vi "Create Init Test Configuration.vi"(8 "error in":errorcluster, 10 "Connection Configuration":T2={"Client?"=FALSE, "Server Certificates"={"Relative Path?"=FALSE, "Certificate Paths"=[], "Certificate Names"=[]}, "Client Certificates"={"Relative Path?"=FALSE, "Certificate Paths"=[], "Certificate Names"=[]}, "Client Configuration"={"Server Endpoint URL"="", "Security Policy"={"Message Mode"=enum."None", "Security"=enum."Basic256"}, "Username/Password"={"Username"="", "Password"=""}}, "Server Configuration"={"Server Name"="", "TCP port (49580)"="49580", "Supported Security Policies"={"None"=TRUE, "Sign with Basic128Rsa125"=FALSE, "Sign and Encrypt with Basic128Rsa125"=FALSE, "Sign with Basic256"=FALSE, "Sign and Encrypt with Basic256"=FALSE}}}) -> (0 "error out":errorcluster, 3 "module":refnum<class "OPC UA configuration.lvclass">)   [LabVIEW 2013, in "OPC UA tests.lvlib"]
doc: "This VI creates the test configuration used in testing. BY default just creates one line with every datatype"
uses:
  OPC UA tests.lvlib
  module/configuration/OPC UA configuration.lvclass
  <vilib>/OPCUA/server/subVI/supported security policies.ctl
  <vilib>/NI/Tag Bus Module Framework/channel/channel classification.ctl
  module/configuration/OPC UA Data Type.ctl
  module/configuration/Line.ctl
  <vilib>/NI/Tag Bus Module Framework/channel/TBM channel.lvclass
  module/configuration/OPC UA configuration.lvclass/OPC UA configuration.ctl
  module/configuration/Write Connection Configuration.vi
  <vilib>/NI/Configuration Framework/serializable configuration/NISE_CEF_serializable configuration.lvclass
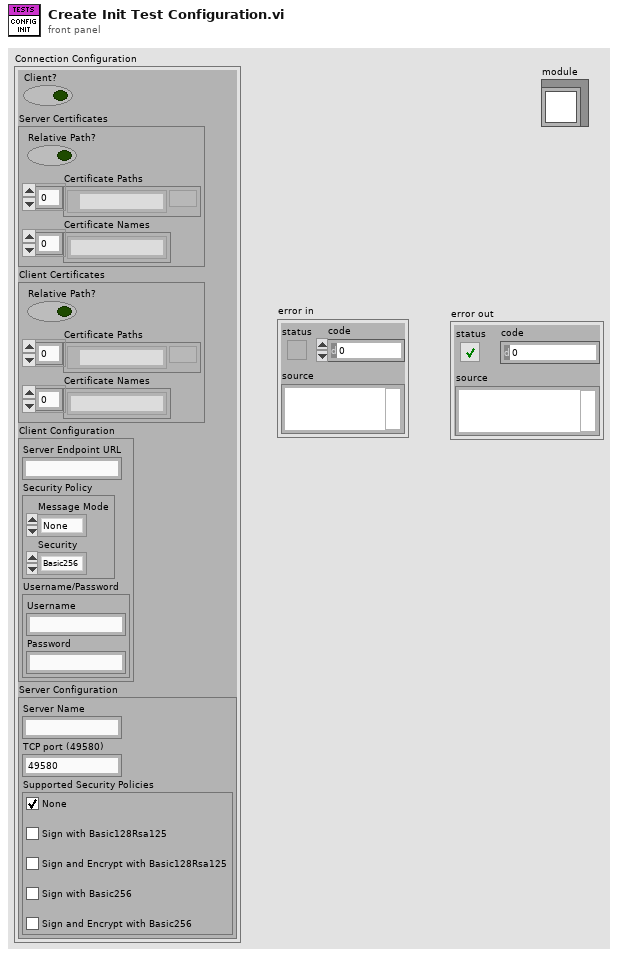
[diagram p1: front panel]
types:
  T1 = typedef "supported security policies.ctl" = cluster{"None":bool, "Sign with Basic128Rsa125":bool, "Sign and Encrypt with Basic128Rsa125":bool, "Sign with Basic256":bool, "Sign and Encrypt with Basic256":bool}
  T2 = cluster{"Client?":bool, "Server Certificates":cluster{"Relative Path?":bool, "Certificate Paths":path[], "Certificate Names":string[]}, "Client Certificates":cluster{"Relative Path?":bool, "Certificate Paths":path[], "Certificate Names":string[]}, "Client Configuration":cluster{"Server Endpoint URL":string, "Security Policy":cluster{"Message Mode":enum16{"None", "Sign", "Sign and Encrypt"}, "Security":enum16{"Basic256", "Basic128Rsa15"}}, "Username/Password":cluster{"Username":string, "Password":string}}, "Server Configuration":cluster{"Server Name":string, "TCP port (49580)":string, "Supported Security Policies":T1}}
  T3 = typedef "TBM channel.lvclass/channel classification.ctl" = enum16{"input data", "output data", "processing parameter", "processing result"}
  T4 = typedef "OPC UA configuration.lvclass/OPC UA Data Type.ctl" = u16
  T5 = typedef "OPC UA configuration.lvclass/Line.ctl" = cluster{"channel":refnum<class "TBM channel.lvclass">, "Node Path":string, "OPC UA Data Type":T4}
  T6 = typedef "tag bus.lvlib/tag descriptor.lvclass/Data Type.ctl" = enum16{"Double", "Single", "I64", "I32", "I16", "I8", "U64", "U32", "U16", "U8", "Boolean", "String", "Array of Double", "Array of Single", "Array of I64", "Array of I32", "Array of I16", "Array of I8", "Array of U64", "Array of U32", "Array of U16", "Array of U8", "Array of Boolean", "Array of String"}
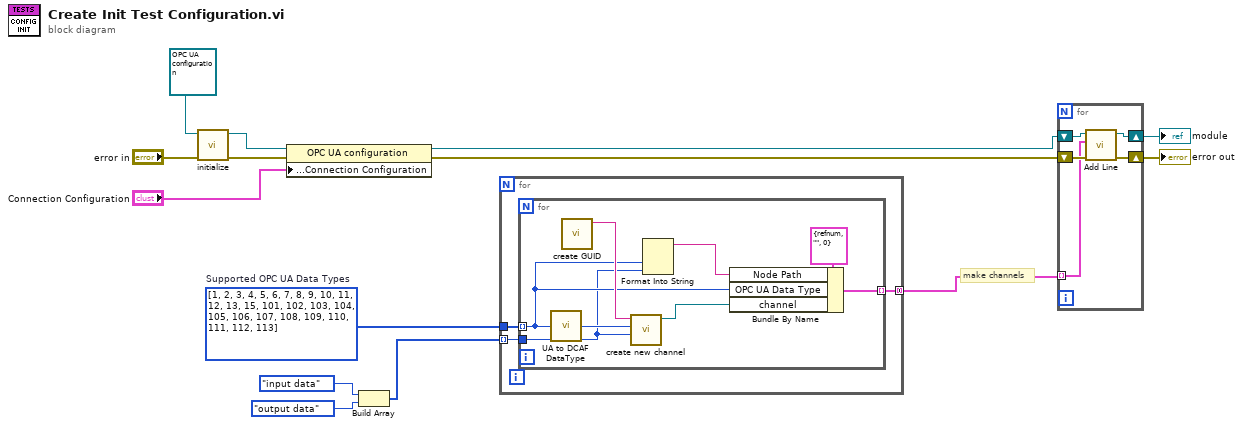
[diagram p0: block diagram]
diagram:
  w5 = T4[] [1, 2, 3, 4, 5, 6, 7, 8, 9, 10, 11, 12, 13, 15, 101, 102, 103, 104, 105, 106, 107, 108, 109, 110, 111, 112, 113] items=["Boolean"=1, "SByte"=2, "Byte"=3, "Int16"=4, "UInt16"=5, "Int32"=6, "UInt32"=7, "Int64"=8, "UInt64"=9, "Float"=10, "Double"=11, "String"=12, "DateTime"=13, "ByteString"=15, "Array of Boolean"=101, "Array of SByte"=102, "Array of Byte"=103, "Array of Int16"=104, "Array of UInt16"=105, "Array of Int32"=106, "Array of UInt32"=107, "Array of Int64"=108, "Array of UInt64"=109, "Array of Float"=110, "Array of Double"=111, "Array of String"=112, "Array of DateTime"=113, "Array of ByteString"=115]  # Supported OPC UA Data Types
  # "make channels"
  n1 = call <vilib>:"initialize.vi"("error in"="error in", "configuration in"=refnum<class "OPC UA configuration.lvclass"> refnum ("tag bus configurable plugin module configuration")) -> ("error out"=w13:errorcluster, "configuration out"=w11:refnum<class "OPC UA configuration.lvclass">)  [unwired: 7 in, 1 out]
  n2 = property class="OPC UA configuration"(reference=w11, error in=w13, "Customize:Properties:Connection Configuration"="Connection Configuration") -> (reference out=w7:refnum<class "OPC UA configuration.lvclass">, error out=w12:errorcluster)
  n3 = Build Array(channel_classification."input data" ("channel classification"), channel_classification."output data" ("channel classification")) -> (w2:T3[])
  n4 = for {
    tunnel: [w17] -> w10 mode=concatenating
    tunnel: w5 -> [w16]
    tunnel: w2 -> [w15] mode=indexing
    n5 = for {
      tunnel: [w23] -> w17 mode=indexing
      tunnel: w16 -> [w19] mode=indexing
      tunnel: w15 -> [w18]
      n6 = call "UA to DCAF DataType.vi"("OPC UA Data Type"=w19) -> ("DCAF Datatype"=w21:T6)
      n7 = call <vilib>:"create GUID.vi"() -> ("uuid"=w25:string)  [unwired: 10 in, 1 out]
      n8 = call <vilib>:"create new channel.vi"("channel classification"=w18, "data type"=w21, "channel name"=w25) -> ("channel"=w22:refnum<class "TBM channel.lvclass">)  [unwired: 8 in]
      n9 = Format Into String(w19, w18) -> (resulting string=w20:string)  [unwired: 3 in, 1 out]
      n10 = Bundle By Name(cluster=T5 {"channel"=refnum, "Node Path"="", "OPC UA Data Type"=0} ("Line"), "Node Path"=w20, "OPC UA Data Type"=w19, "channel"=w22) -> (w23:T5)
    }
  }
  n11 = for {
    tunnel: w10 -> [w26] mode=indexing
    shift-right: [w29] -> w9
    shift-left: w7 -> [w30]
    shift-right: [w27] -> w14
    shift-left: w12 -> [w28]
    n12 = call "Add Line.vi"("error in"=w28, "Line"=w26, "OPC UA configuration in"=w30) -> ("error out"=w27:errorcluster, "OPC UA configuration out"=w29:refnum<class "OPC UA configuration.lvclass">)  [unwired: 7 in]
  }
  "error out" <- w14
  "module" <- w9
